vi "LatchOpen.vi"   [LabVIEW 2014, in "LatchLib.lvlib"]
uses:
  LatchLib.lvlib
  LatchRefs.ctl
  <vilib>/Rock Robotics/WPI/Solenoid/WPI_SolenoidChannel.ctl
  <vilib>/Rock Robotics/WPI/Solenoid/WPI_SolenoidOpenDouble.vi
types:
  T1 = typedef "WPI_SolenoidChannel.ctl" = enum8{"Solenoid 0", "Solenoid 1", "Solenoid 2", "Solenoid 3", "Solenoid 4", "Solenoid 5", "Solenoid 6", "Solenoid 7", "Invalid"}
  T2 = typedef "LatchLib.lvlib/LatchRefs.ctl" = enum16{"LatchSloenoid", "ContainerSolenoid"}
  T3 = typedef "WPI_SolenoidDevRef.ctl" = cluster{"DevStatus":errorcluster, "Pneumatics Control Module":u8, "Forward Solenoid Channel":T1, "Reverse Solenoid Channel":T1}
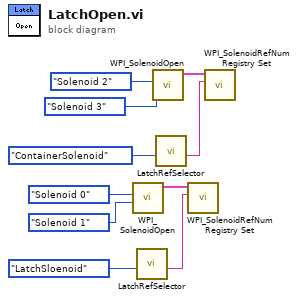
[diagram p0: block diagram]
diagram:
  n1 = call-poly <vilib>:"WPI_SolenoidOpen.vi"("Reverse Solenoid Channel"=WPI_SolenoidChannel."Solenoid 1", "Forward Solenoid Channel"=WPI_SolenoidChannel."Solenoid 0") -> ("SolenoidDevRef"=w9:T3)  [unwired: 8 in, 1 out]
  n2 = call "LatchRefSelector.vi"("Enum"=LatchRefs."LatchSloenoid") -> ("String"=w10:string)  [unwired: 10 in]
  n3 = call-poly <vilib>:"WPI_SolenoidOpen.vi"("Reverse Solenoid Channel"=WPI_SolenoidChannel."Solenoid 3", "Forward Solenoid Channel"=WPI_SolenoidChannel."Solenoid 2" ("Solenoid Channel")) -> ("SolenoidDevRef"=w7:T3)  [unwired: 8 in, 1 out]
  n4 = call "LatchRefSelector.vi"("Enum"=LatchRefs."ContainerSolenoid") -> ("String"=w8:string)  [unwired: 10 in]
  n5 = call <vilib>:"WPI_SolenoidRefNum Registry Set.vi"("refnum name"=w10, "SolenoidDevRef"=w9) -> ()  [unwired: 8 in, 2 out]
  n6 = call <vilib>:"WPI_SolenoidRefNum Registry Set.vi"("refnum name"=w8, "SolenoidDevRef"=w7) -> ()  [unwired: 8 in, 2 out]
